vi "Get Channel Data in Section.vi"(6 "Get FIFO indexes (T)":bool=TRUE, 7 "Custom device ref":T1 format="%.0x", 8 "error in (no error)":errorcluster, 9 "Channels":string[](array[string]), 10 "Section (\"\":none)":string, 11 "Item Ref in":T1 format="%.0x") -> (0 "error out":errorcluster, 1 "default values":dbl[](array[numeric]), 2 "FIFO indexes":i32[](array[numeric]), 3 "Item Ref out":T1 format="%.0x", 5 "channel refs":T1[](array[typedef]) format="%.0x")   [LabVIEW 2013, in "Engine Simulation Toolkit System Explorer.lvlib"]
uses:
  Engine Simulation Toolkit System Explorer.lvlib
  <vilib>/NI Veristand/Custom Device API/Custom Device Item Ref.ctl
  <vilib>/NI Veristand/Custom Device API/Custom Device API.lvlib
  <vilib>/NI Veristand/Custom Device Tools/Custom Device Utility Library/Custom Device Utility Library.lvlib
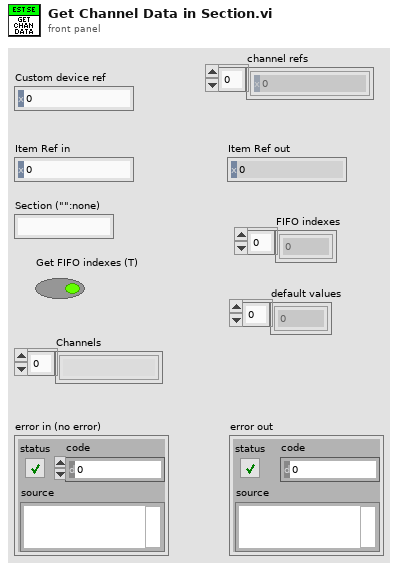
[diagram p1: front panel]
types:
  T1 = typedef "Custom Device API.lvlib/Custom Device Item Ref.ctl" = u64
  T2 = typedef "Custom Device API.lvlib/Custom Device Channel.ctl" = cluster{"Type":T3, "Units":string, "Default Value":dbl, "Faultable":bool, "Scalable":bool}
  T3 = typedef "Custom Device API.lvlib/Custom Device Channel Type.ctl" = enum16{"Input", "Output"}
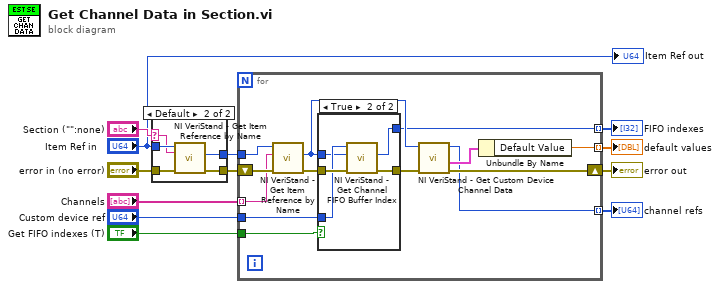
[diagram p0: block diagram]
diagram:
  n1 = case shown="Default" "Section (\"\":none)" {
    selector: "Section (\"\":none)" -> [_ w15]
    tunnel: [w14 w19] -> w9
    tunnel: [w13 w18] -> w8
    tunnel: "Item Ref in" -> [w14 w17]
    tunnel: "error in (no error)" -> [w13 w16]
    frame "" {
    }
    frame Default {
      n2 = call <vilib>:"NI VeriStand - Get Item Reference by Name.vi"("error in (no error)"=w16, "Item Name"=w15, "Parent Ref in"=w17) -> ("error out"=w18:errorcluster, "Item Ref"=w19:T1)  [unwired: 5 in, 2 out]
    }
  }
  n3 = for {
    shift-right: [w28] -> w11
    shift-left: w8 -> [w32]
    tunnel: w9 -> [w31]
    tunnel: "Channels" -> [w30] mode=indexing
    tunnel: [w26] -> w12 mode=indexing
    tunnel: "Custom device ref" -> [w24]
    tunnel: [w22] -> w3 mode=indexing
    tunnel: "Get FIFO indexes (T)" -> [w21]
    tunnel: [w20] -> w1 mode=indexing
    n4 = call <vilib>:"NI VeriStand - Get Item Reference by Name.vi"("error in (no error)"=w32, "Item Name"=w30, "Parent Ref in"=w31) -> ("error out"=w29:errorcluster, "Item Ref"=w23:T1)  [unwired: 5 in, 2 out]
    n5 = case shown="True" w21 {
      tunnel: w29 -> [w33 w38]
      tunnel: [w33 w37] -> w25
      tunnel: w24 -> [_ w36]
      tunnel: w23 -> [_ w35]
      tunnel: [_ w34] -> w22
      frame False {
      }
      frame True {
        n6 = call <vilib>:"NI VeriStand - Get Channel FIFO Buffer Index.vi"("error in"=w38, "Channel Ref"=w35, "Device Ref in"=w36) -> ("error out"=w37:errorcluster, "Channel FIFO Buffer Index"=w34:i32)  [unwired: 4 in, 3 out]
      }
    }
    n7 = call <vilib>:"NI VeriStand - Get Custom Device Channel Data.vi"("error in (no error)"=w25, "Channel Ref in"=w23) -> ("error out"=w28:errorcluster, "Channel"=w27:T2, "Channel Ref out"=w20:T1)  [unwired: 4 in, 3 out]
    n8 = Unbundle By Name(w27) -> ("Default Value"=w26:dbl)
  }
  "default values" <- w12
  "error out" <- w11
  "FIFO indexes" <- w3
  "channel refs" <- w1
  "Item Ref out" <- "Item Ref in"
